vi "Send Interface Status.vi"(8 "error in (no error)":errorcluster, 10 "Message":string, 11 "Stream in":refnum<class "Stream.lvclass">) -> (0 "error out":errorcluster, 3 "Stream out":refnum<class "Stream.lvclass">)   [LabVIEW 2018, in "Stream.lvclass"]
uses:
  Stream.lvclass
  Stream.lvclass/Stream.ctl
  Interface/Interface.lvclass/Interface.ctl
  Interface/Interface.lvclass
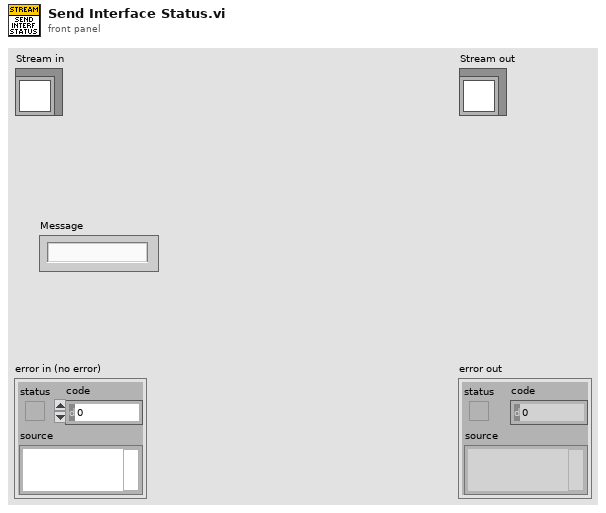
[diagram p1: front panel]
types:
  T1 = cluster{"Current Temperature":i16, "Temperatue Status":string}
  T2 = cluster{"Initialization":bool, "Serial Number":u16}
  T3 = cluster{"Exposure Time":sgl, "Pre-amp gain":u8, "Readout Rate":u8, "EM Mode":u8, "EM Gain":u16, "Binning":u16, "Initial Line":u16, "Initial Cloumn":u16, "Final Line":u16, "Final Column":u16, "Kinetic Series Length":u32, "Shutter Mode":u8, "Cooler ON/OFF":u16, "Temperature":i8, "Image Name":string, "Image Path":string, "#Images":u32, "#index":u16}
  T4 = cluster{"Current Exptime":sgl, "Exposures Done":u16, "Last Image":string, "Disk Space":u16, "Exptime":sgl, "NImages":u16, "#index":u16, "File Base Name":string, "Image Path":string, "OBS Title":string, "Comment":string, "DS9":bool, "Cam_Status":string}
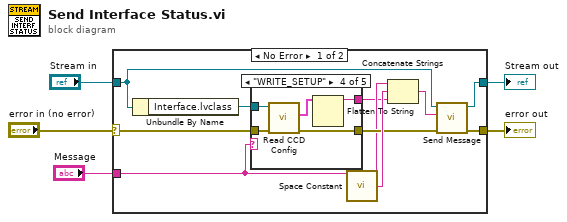
[diagram p0: block diagram]
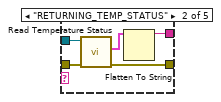
[diagram p3: hidden frame]
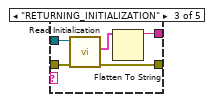
[diagram p4: hidden frame]
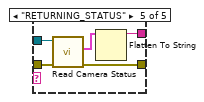
[diagram p5: hidden frame]
diagram:
  n1 = case shown="No Error" "error in (no error)" {
    selector: "error in (no error)" -> [w8 w38]
    tunnel: [w13 w38] -> w4
    tunnel: [w10 w37] -> w2
    tunnel: "Stream in" -> [w11 w37]
    tunnel: "Message" -> [w7 _]
    frame No Error {
      n2 = Unbundle By Name(w11) -> ("Interface.lvclass"=w15:refnum<class "Interface.lvclass">)
      n3 = case shown="\"WRITE_SETUP\"" w7 {
        tunnel: w15 -> [_ w21 w26 w28 w33]
        tunnel: [w16 w20 w25 w29 w34] -> w9
        tunnel: w8 -> [w16 w19 w24 w30 w35]
        tunnel: [_ w17 w22 w31 w36] -> w6
        frame "False", Default {
        }
        frame "RETURNING_TEMP_STATUS" {
          n4 = call "Read Temperature Status.vi"("error in (no error)"=w19, "Interface in"=w21) -> ("error out"=w20:errorcluster, "Temperature Status"=w18:T1)  [unwired: 7 in, 1 out]
          n5 = Flatten To String(anything=w18) -> (data string=w17:string)  [unwired: 3 in, 2 out]
        }
        frame "RETURNING_INITIALIZATION" {
          n6 = call "Read Initialization.vi"("error in (no error)"=w24, "Interface in"=w26) -> ("error out"=w25:errorcluster, "Initialization"=w23:T2)  [unwired: 7 in, 1 out]
          n7 = Flatten To String(anything=w23) -> (data string=w22:string)  [unwired: 3 in, 2 out]
        }
        frame "WRITE_SETUP" {
          n8 = call "Read CCD Config.vi"("error in (no error)"=w30, "Interface in"=w28) -> ("error out"=w29:errorcluster, "CCD Config"=w27:T3)  [unwired: 7 in, 1 out]
          n9 = Flatten To String(anything=w27) -> (data string=w31:string)  [unwired: 3 in, 2 out]
        }
        frame "RETURNING_STATUS" {
          n10 = call "Read Camera Status.vi"("error in (no error)"=w35, "Interface in"=w33) -> ("error out"=w34:errorcluster, "Camera Status"=w32:T4)  [unwired: 7 in, 1 out]
          n11 = Flatten To String(anything=w32) -> (data string=w36:string)  [unwired: 3 in, 2 out]
        }
      }
      n12 = call <vilib>:"Space Constant.vi"() -> ("String"=w14:string)
      n13 = Concatenate Strings(w7, w14, w6) -> (w12:string)
      n14 = call "Send Message.vi"("error in (no error)"=w9, "Message"=w12, "Stream in"=w11) -> ("error out"=w13:errorcluster, "Stream out"=w10:refnum<class "Stream.lvclass">)  [unwired: 7 in]
    }
    frame Error {
    }
  }
  "error out" <- w4
  "Stream out" <- w2
